vi "temperatura.vi"() -> ()   [LabVIEW 2025]
uses:
  <vilib>/Instr/_visa.llb/VISA Configure Serial Port (Instr).vi
panel:
  out "Boolean":bool
  out "read buffer":string
  out "Gauge":dbl(knob) scale=0.0..100.0
  out "Thermometer":dbl(slide) scale=0.0..100.0
  in  "stop":bool
  in  "VISA resource name":refnum<visa-resource-name>
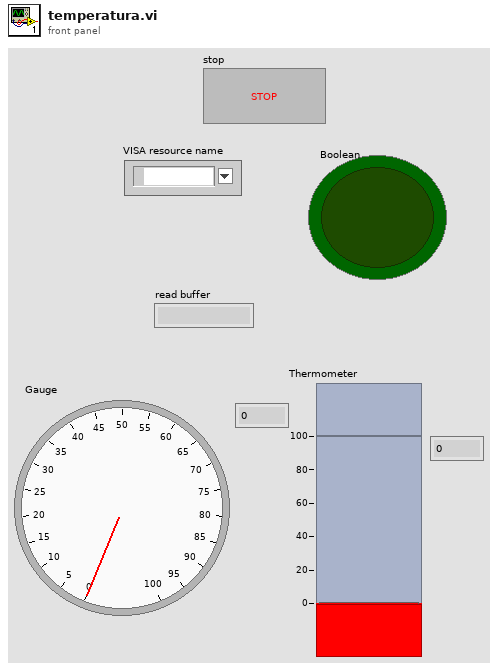
[diagram p1: front panel]
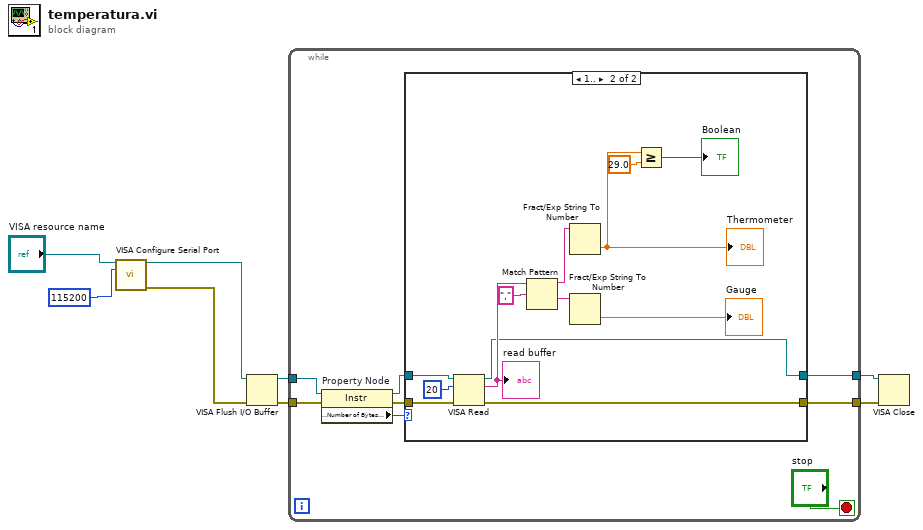
[diagram p0: block diagram]
diagram:
  n1 = call-poly "VISA Configure Serial Port"("VISA resource name"="VISA resource name", "baud rate (9600)"=u32 115200) -> ("VISA resource name out"=w7:refnum<visa-resource-name>, "error out"=w6:errorcluster)  [unwired: 12 in]
  n2 = VISA Flush I/O Buffer(VISA resource name=w7, error in (no error)=w6) -> (VISA resource name out=w5:refnum<visa-resource-name>, error out=w4:errorcluster)  [unwired: 1 in]
  n3 = while {
    tunnel: w5 -> [w16]
    tunnel: w4 -> [w15]
    tunnel: [w10] -> w3
    tunnel: [w9] -> w2
    stop <- "stop" stop-if-true
    n4 = property on="Property Node" class="Instr"(reference=w16, error in=w15) -> (reference out=w14:refnum<visa-resource-name>, error out=w13:errorcluster, "Serial Settings:Number of Bytes at Serial Port"=w11:u32)
    n5 = case shown="1.." w11 {
      tunnel: w14 -> [w18 w31]
      tunnel: w13 -> [w17 w30]
      tunnel: [w17 w27] -> w10
      tunnel: [w18 w26] -> w9
      frame 0, Default {
      }
      frame 1.. {
        n6 = VISA Read(VISA resource name=w31, byte count=u32 20, error in (no error)=w30) -> (VISA resource name out=w26:refnum<visa-resource-name>, read buffer=w29:string, error out=w27:errorcluster)  [unwired: 1 out]
        "read buffer" <- w29
        n7 = Match Pattern(string=w29, regular expression=",") -> (before substring=w25:string, after substring=w24:string)  [unwired: 1 in, 2 out]
        n8 = Fract/Exp String To Number(string=w25) -> (number=w21:dbl)  [unwired: 3 in, 1 out]
        "Thermometer" <- w21
        n9 = Fract/Exp String To Number(string=w24) -> (number=→"Gauge":dbl)  [unwired: 3 in, 1 out]
        n10 = Greater Or Equal?(x=w21, y=29.0) -> (x >= y?=→"Boolean":bool)
      }
    }
  }
  n11 = VISA Close(VISA resource name=w2, error in (no error)=w3) -> ()  [unwired: 1 out]
